vi "SendCommand.vi"(8 "error in (no error)":errorcluster, 10 "command":string="c\r", 11 "Serial Controller in":refnum<class "Serial Controller.lvclass">) -> (0 "error out":errorcluster, 2 "Returned":string, 3 "Serial Controller out":refnum<class "Serial Controller.lvclass">)   [LabVIEW 2012, in "Serial Controller.lvclass"]
uses:
  Serial Controller.lvclass
  Serial Controller.lvclass/Serial Controller.ctl
panel:
  out "return count":u32
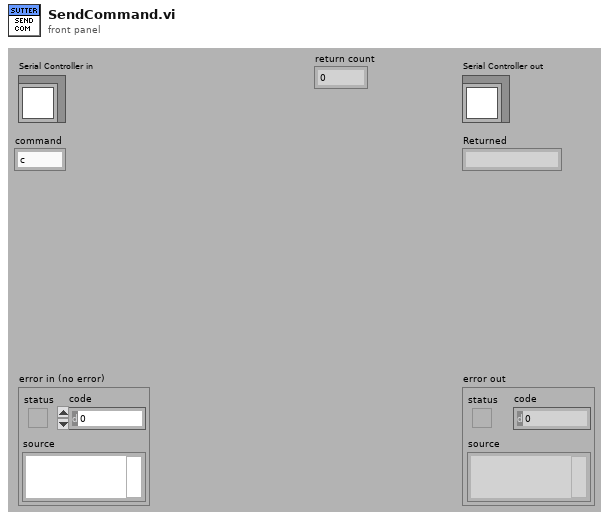
[diagram p1: front panel]
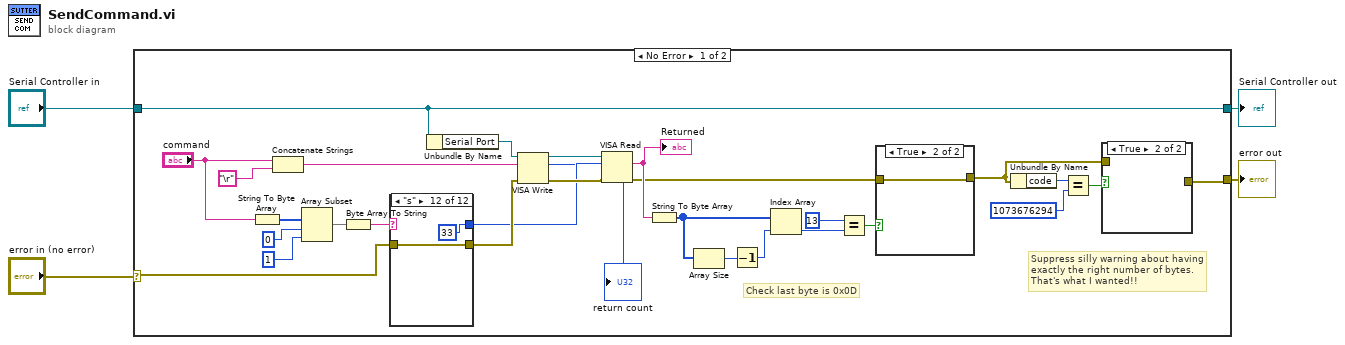
[diagram p0: block diagram]
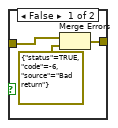
[diagram p3: hidden frame]
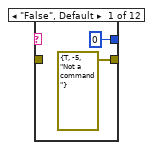
[diagram p4: hidden frame]
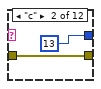
[diagram p5: hidden frame]
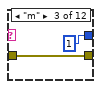
[diagram p6: hidden frame]
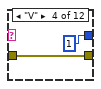
[diagram p7: hidden frame]
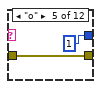
[diagram p8: hidden frame]
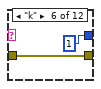
[diagram p9: hidden frame]
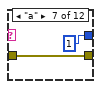
[diagram p10: hidden frame]
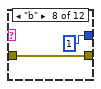
[diagram p11: hidden frame]
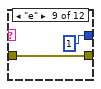
[diagram p12: hidden frame]
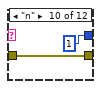
[diagram p13: hidden frame]
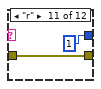
[diagram p14: hidden frame]
diagram:
  n1 = case shown="No Error" "error in (no error)" {
    selector: "error in (no error)" -> [w23 w64]
    tunnel: [w8 w64] -> w3
    tunnel: [w30 w63] -> w1
    tunnel: "Serial Controller in" -> [w30 w63]
    frame No Error {
      # "Check last byte is 0x0D"
      # "Suppress silly warning about having \nexactly the right number of bytes. \nThat's what I wanted!!"
      n2 = String To Byte Array(string="command") -> (unsigned byte array=w28:u8[])
      n3 = Concatenate Strings("command", "\r" ("write buffer")) -> (w21:string)
      n4 = Array Subset(array=w28, index=0, length=1) -> (w25:u8[])
      n5 = Byte Array To String(unsigned byte array=w25) -> (string=w24:string)
      n6 = case shown="\"s\"" w24 {
        tunnel: [0 13 1 1 1 1 1 1 1 1 1 33] -> w7
        tunnel: w23 -> [_ w41 w43 w45 w47 w49 w51 w53 w55 w57 w59 w61]
        tunnel: [errorcluster {"status"=TRUE, "code"=-5, "source"="Not a command"} ("error IO") w41 w43 w45 w47 w49 w51 w53 w55 w57 w59 w61] -> w22
        frame "False", Default {
        }
        frame "c" {
        }
        frame "m" {
        }
        frame "V" {
        }
        frame "o" {
        }
        frame "k" {
        }
        frame "a" {
        }
        frame "b" {
        }
        frame "e" {
        }
        frame "n" {
        }
        frame "r" {
        }
        frame "s" {
        }
      }
      n7 = Unbundle By Name(w30) -> ("Serial Port"=w33:refnum<visa-resource-name>)
      n8 = VISA Write(VISA resource name=w33, write buffer=w21, error in (no error)=w22) -> (VISA resource name out=w32:refnum<visa-resource-name>, return count=→"return count":u32, error out=w31:errorcluster)
      n9 = VISA Read(VISA resource name=w32, byte count=w7, error in (no error)=w31) -> (read buffer=w20:string, error out=w12:errorcluster)  [unwired: 2 out]
      "Returned" <- w20
      n10 = String To Byte Array(string=w20) -> (unsigned byte array=w18:u8[])
      n11 = Array Size(array=w18) -> (size(s)=w17:i32)
      n12 = Decrement(x=w17) -> (x-1=w16:i32)
      n13 = Index Array(array=w18, index=w16) -> (element=w15:u8)
      n14 = Equal?(x=u8 13, y=w15) -> (x = y?=w13:bool)
      n15 = case shown="True" w13 {
        tunnel: w12 -> [w37 w38]
        tunnel: [w35 w38] -> w5
        frame False {
          n16 = Merge Errors(w37, errorcluster {"status"=TRUE, "code"=-6, "source"="Bad return"} ("error out")) -> (w35:errorcluster)
        }
        frame True {
        }
      }
      n17 = Unbundle By Name(w5) -> ("code"=w11:i32)
      n18 = Equal?(x=w11, y=1073676294) -> (x = y?=w9:bool)
      n19 = case shown="True" w9 {
        tunnel: w5 -> [w34 _]
        tunnel: [w34 _] -> w8
        frame False {
        }
        frame True {
        }
      }
    }
    frame Error {
    }
  }
  "error out" <- w3
  "Serial Controller out" <- w1
